vi "Find Component Center.vi"() -> ()   [LabVIEW 2019]
uses:
  Classes/Workspace/Workspace.ctl
  Classes/Workspace/Component/Component Tray.lvclass
  Classes/Controller/Controller.lvclass
  Classes/Workspace/Fixture.lvclass
panel:
  out "error out":errorcluster
  out "Workspace":T1
  in  "error in (no error)":errorcluster
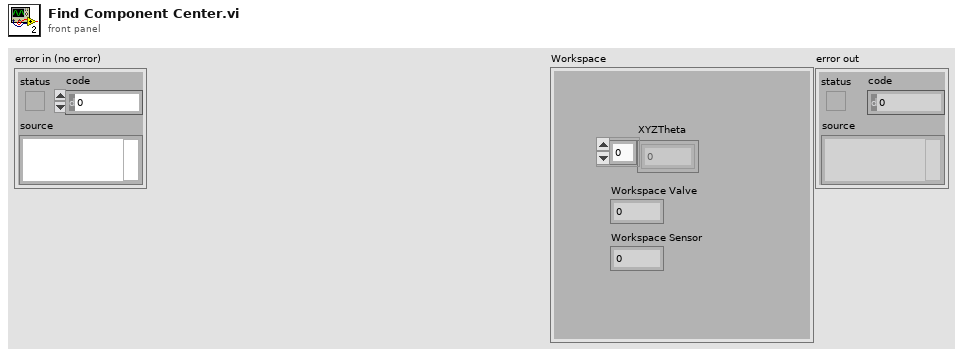
[diagram p1: front panel]
types:
  T1 = typedef "Fixture.lvclass/Workspace.ctl" = cluster{"XYZTheta":dbl[], "Workspace Valve":i32, "Workspace Sensor":i32}
  T2 = typedef "Controller.lvclass/Controllers.ctl" = cluster{"I-O.lvclass":refnum<class "I-O.lvclass">, "Dispenser.lvclass":refnum<class "Dispenser.lvclass">, "Gantry":refnum<k24>}
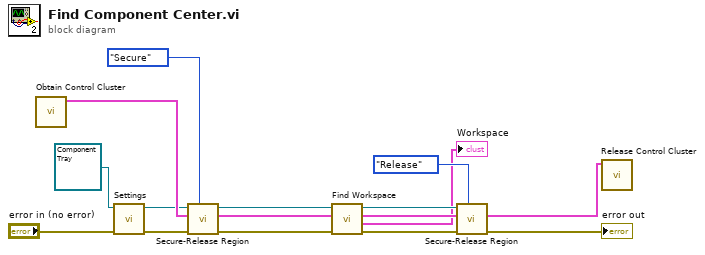
[diagram p0: block diagram]
diagram:
  n1 = call "Obtain Control Cluster.vi"() -> ("Control Out"=w14:T2)  [unwired: 11 in]
  n2 = call-dynamic "Settings.vi"("error in (no error)"="error in (no error)", "Component in"=refnum<class "Component Tray.lvclass"> refnum ("Component Tray.lvclass")) -> ("error out"=w12:errorcluster, "Component out"=w13:refnum<class "Component Tray.lvclass">)  [unwired: 8 in]
  n3 = call-dynamic "Secure-Release Region.vi"("Action"=enum16{"Secure", "Release"}."Secure", "error in (no error)"=w12, "Control In"=w14, "Workspace in"=w13) -> ("error out"=w8:errorcluster, "Control Out"=w9:T2, "Workspace out"=w10:refnum<class "Component Tray.lvclass">)  [unwired: 5 in]
  n4 = call-dynamic "Find Workspace.vi"("error in (no error)"=w8, "Control In"=w9, "Component.lvclass"=w10) -> ("error out"=w3:errorcluster, "Workspace"=→"Workspace":T1, "Control Out"=w5:T2, "Workspace Out"=w6:refnum<class "Component Tray.lvclass">)  [unwired: 5 in]
  n5 = call-dynamic "Secure-Release Region.vi"("Action"=enum16{"Secure", "Release"}."Release", "error in (no error)"=w3, "Control In"=w5, "Workspace in"=w6) -> ("error out"=→"error out":errorcluster, "Control Out"=w2:T2)  [unwired: 5 in, 1 out]
  n6 = call "Release Control Cluster.vi"("output cluster"=w2) -> ()  [unwired: 11 in]
